vi "Method.vi"(4 "Value":refnum<class "Abs_Double Float.lvclass">) -> (1 "Result":refnum<class "Abs_Double Float.lvclass">)   [LabVIEW 2021, in "Decrement_DBL.lvclass"]
uses:
  Decrement_DBL.lvclass
  Abs_Types/Double Float/Abs_Double Float.lvclass
  C:/Users/Tim/Documents/LabVIEW/2021/Data Classes/Source/Functions/Support/One Terminal/DBL/AbsFunc_One Term_DBL.lvclass
  C:/Users/Tim/Documents/LabVIEW/2021/Data Classes/Source/Abs_Types/Double Float/Abs_Double Float.lvclass
  Support/One Terminal/DBL/AbsFunc_One Term_DBL.lvclass/AbsFunc_One Term_DBL.ctl
  Support/One Terminal/DBL/Properties/Write Numeric A.vi
  Decrement_DBL.lvclass/Decrement_DBL.ctl
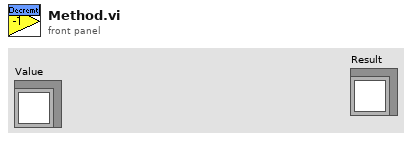
[diagram p1: front panel]
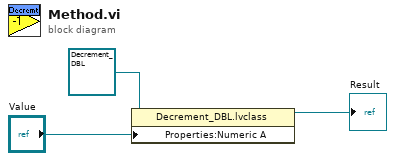
[diagram p0: block diagram]
diagram:
  n1 = property class="Decrement_DBL.lvclass"(reference=refnum<class "Decrement_DBL.lvclass"> refnum ("Decrement_DBL.lvclass"), "Properties:Numeric A"="Value") -> (reference out=→"Result":refnum<class "Decrement_DBL.lvclass">)  [unwired: 1 in, 1 out]
